vi "Waveform Processing Hub.vi"() -> ()   [LabVIEW 2014]
uses:
  <vilib>/Utility/file.llb/Write To Spreadsheet File (DBL).vi
  <vilib>/Utility/file.llb/Read From Spreadsheet File (DBL).vi
panel:
  in  "Baseline Pinch":bool
  in  "Orthogonal String Array Cluster":cluster{"Orthogonal String Array":string[]}={"Orthogonal String Array"=["1.1", "1.3", "1.5", "2.2", "2.4", "2.6", "2.8", "3.1", "3.3", "3.5", "3.7", "3.9", "4.4", "5.5", "6.8"]}
  in  "Empty String Array Cluster":cluster{"Empty String Array":string[]}
  in  "2-45 String Array Cluster":cluster{"2-45 String Array":string[]}={"2-45 String Array"=["2", "3", "4", "5", "6", "7", "8", "9", "10", "11", "12", "13", "14", "15", "16", "17", "18", "19", "20", "21", "22", "23", "24", "25", "26", "27", "28", "29", "30", "31", "32", "33", "34", "35", "36", "37", "38", "39", "40", "41", "42", "43", "44", "45"]}
  in  "1-5 String Array Cluster":cluster{"1-5 String Array":string[]}={"1-5 String Array"=["1", "2", "3", "4", "5"]}
  out "wfilter family":string="sym"
  out "MATLAB wfliter":string="sym5"
  out "Program Iterations":i32
  in  "Tab Control":T1(tab)
  out "Vertical Indicator":bool
  in  "Flip Vertically button":bool
  out "Horizontal Indicator":bool
  in  "Flip Horizontally Button":bool
  in  "Select File Type":string(combo)="Tab Delimited"
  out "Loaded File Data":dbl[][](graph)
  out "File Data":dbl[][](array[numeric])
  in  "Open Button":bool
  in  "Transpose":bool
  out "Transpose Indicator":bool
  out "Filtering Progress":u8(slide) scale=0.0..100.0
  out "Processed Spectra":dbl[][](graph)
  in  "Zero Data":bool
  in  "Normalize Data":bool
  out "File Data":dbl[][](graph)
  in  "Savitzy-Golay Filter":bool
  in  "Polynomial Order":i32=9
  in  "Side Points":i32=7
  in  "Play Button":bool
  in  "DWT BG Remove":bool
  in  "BG Remove Iterations":dbl=10.0
  in  "Wavelet #":string(combo)="5"
  in  "Wavelet Family":string(combo)="Symlets"
  in  "Process Spectra Separately":bool
  in  "Scale [>0]":dbl=8.0
  in  "DWT Filter":bool
  in  "# H-Freq Cuts":dbl=1.0
  in  "# L-Freq Cuts":dbl
  out "Zero & Normalized Data Out":dbl[][](array[numeric])
  in  "Save Button":bool
  out "File Data 2":dbl[][](graph)
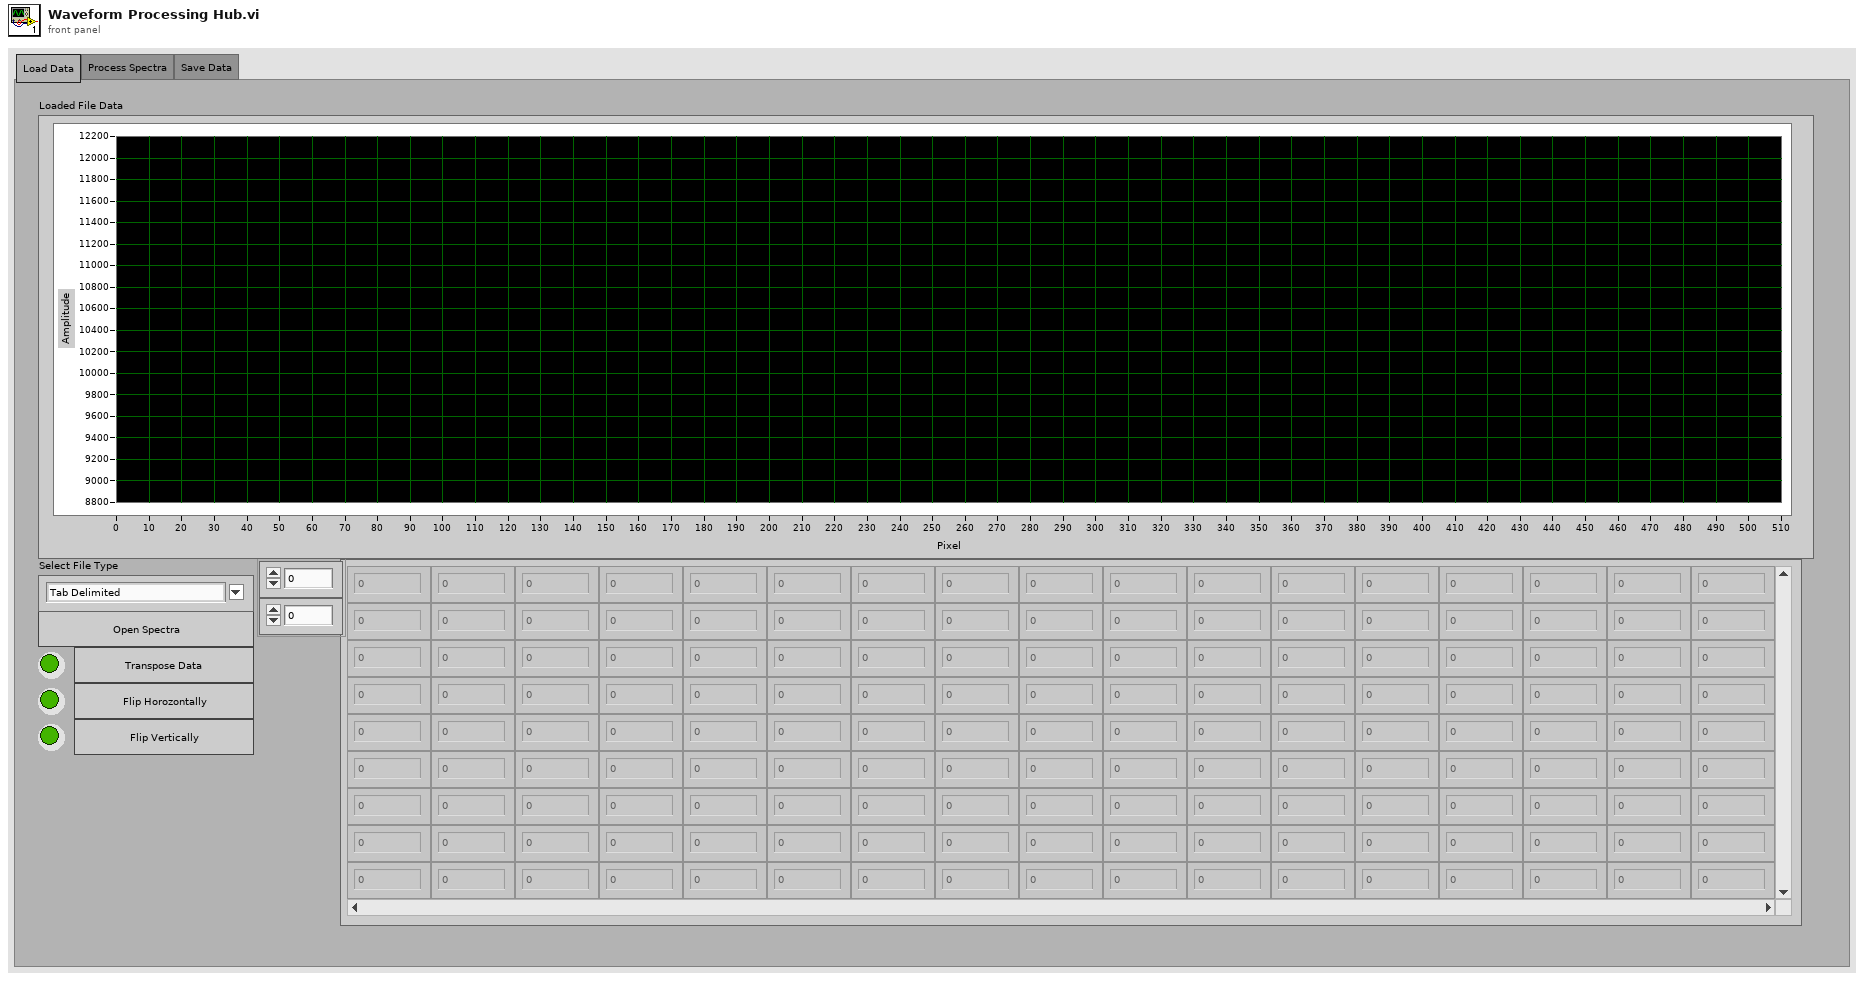
[diagram p1: front panel]
types:
  T1 = enum32{"Load Data", "Process Spectra", "Save Data"}
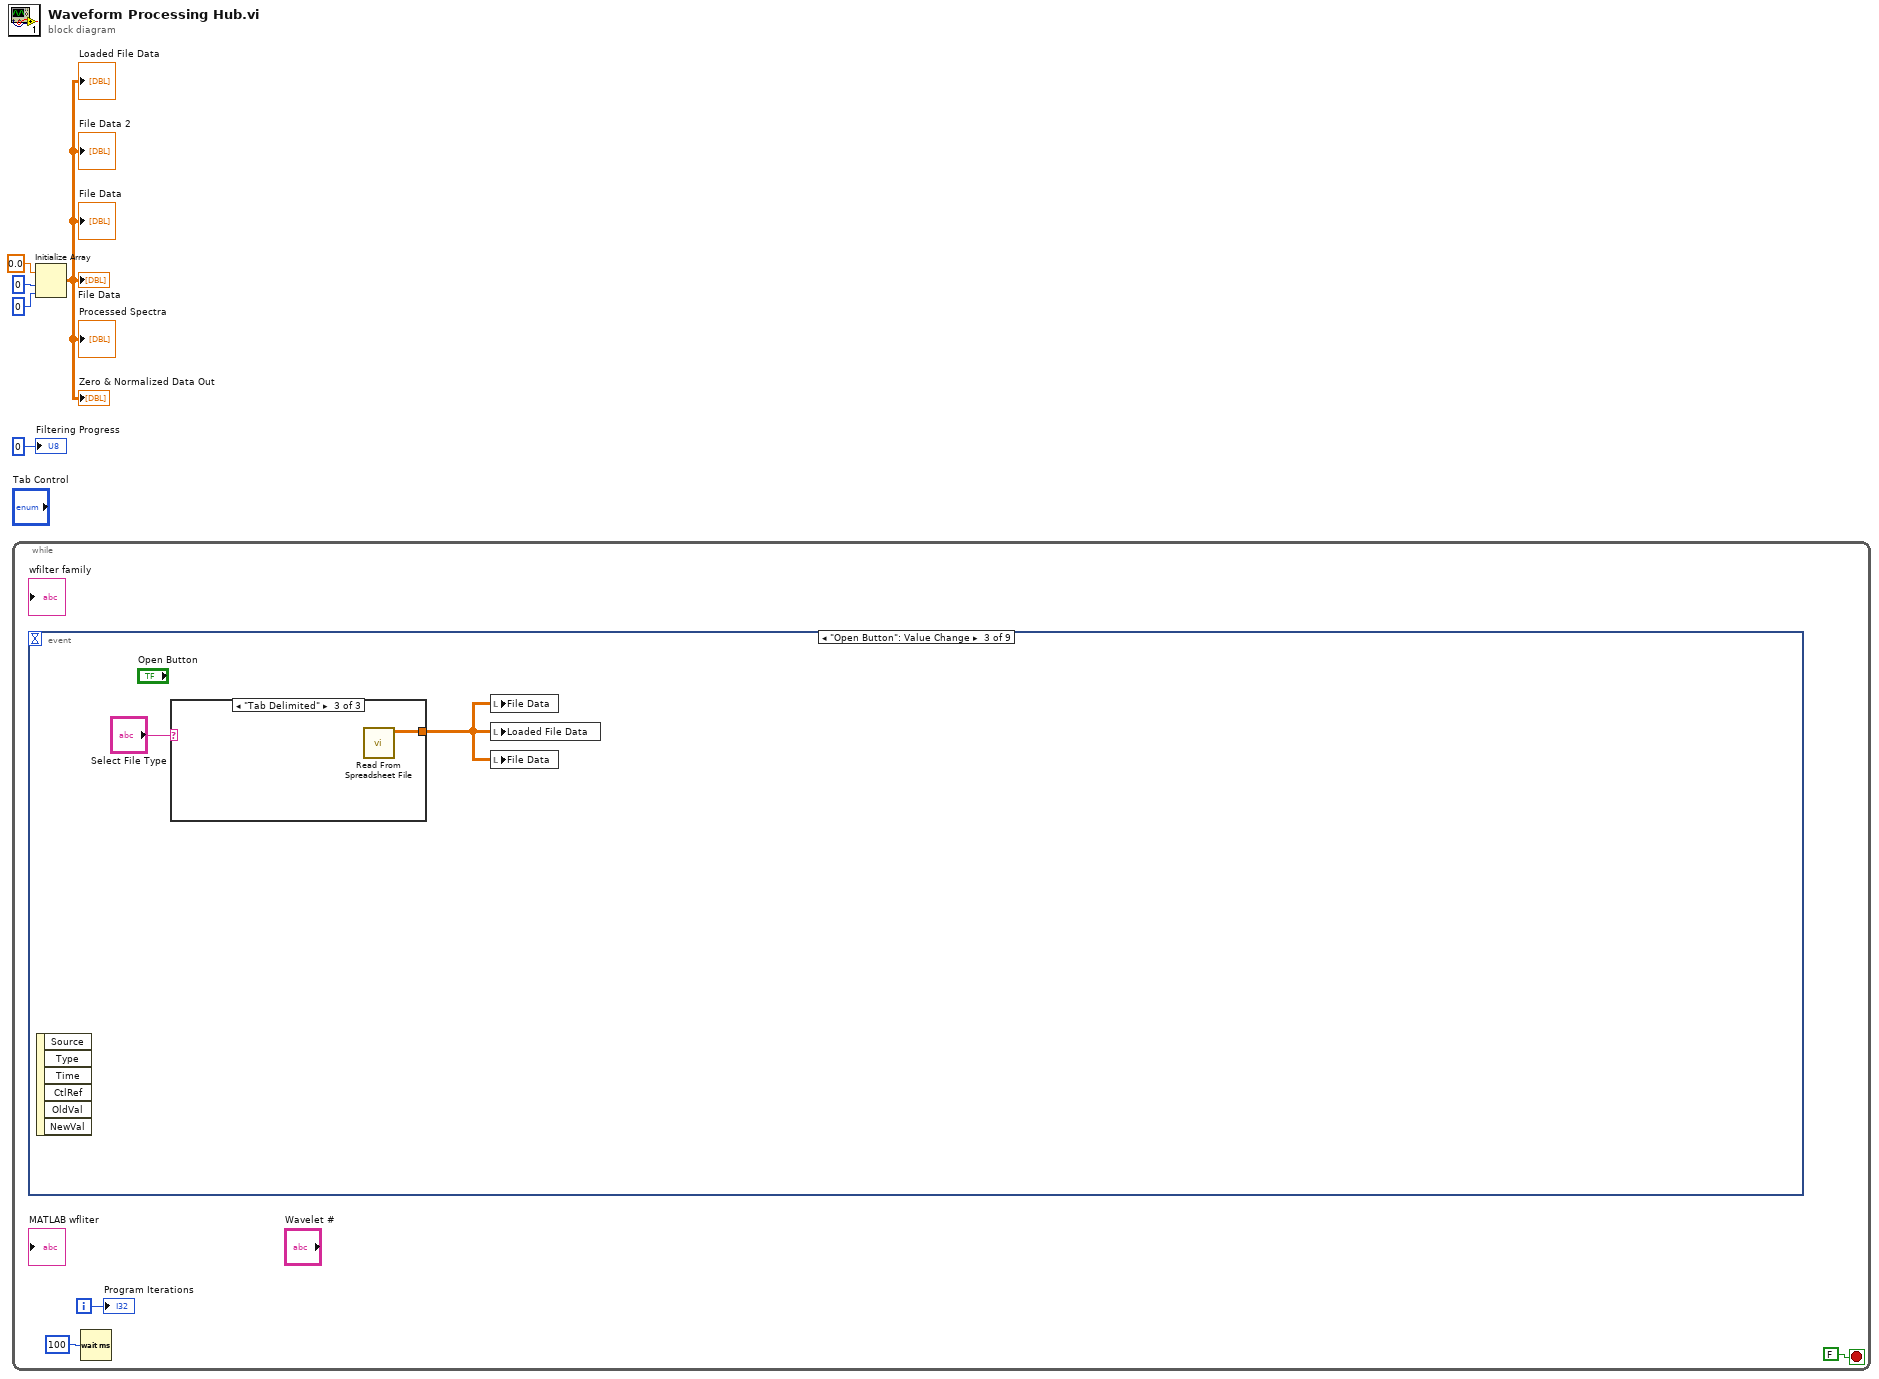
[diagram p0: block diagram]
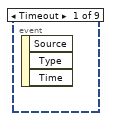
[diagram p2: hidden frame]
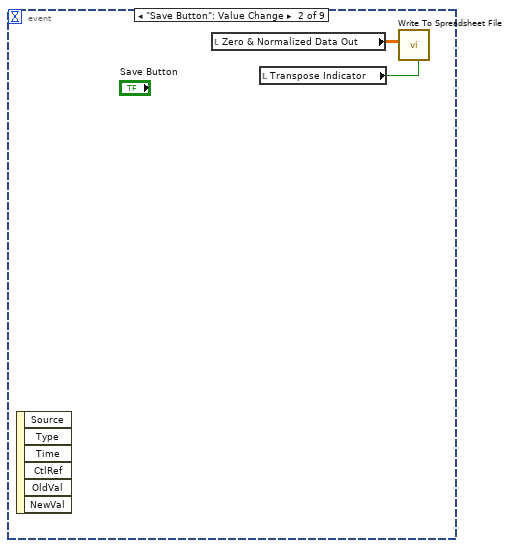
[diagram p3: hidden frame]
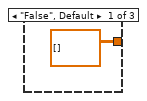
[diagram p4: hidden frame]
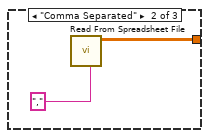
[diagram p5: hidden frame]
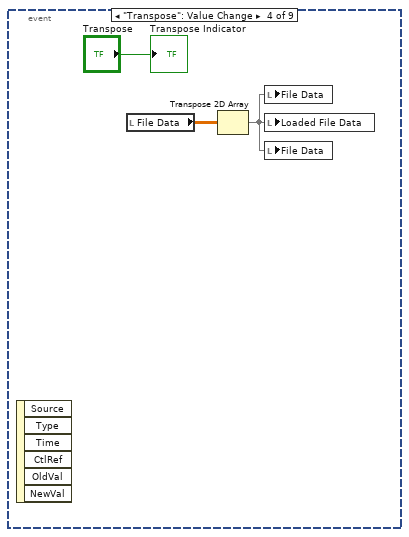
[diagram p6: hidden frame]
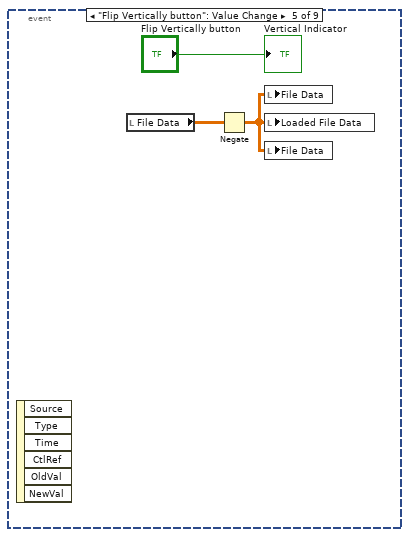
[diagram p7: hidden frame]
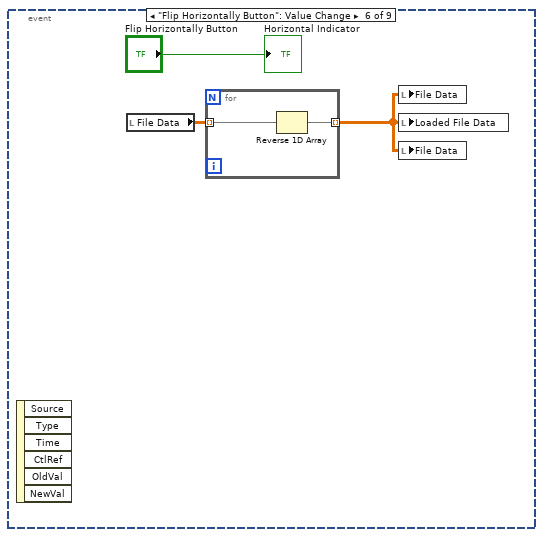
[diagram p8: hidden frame]
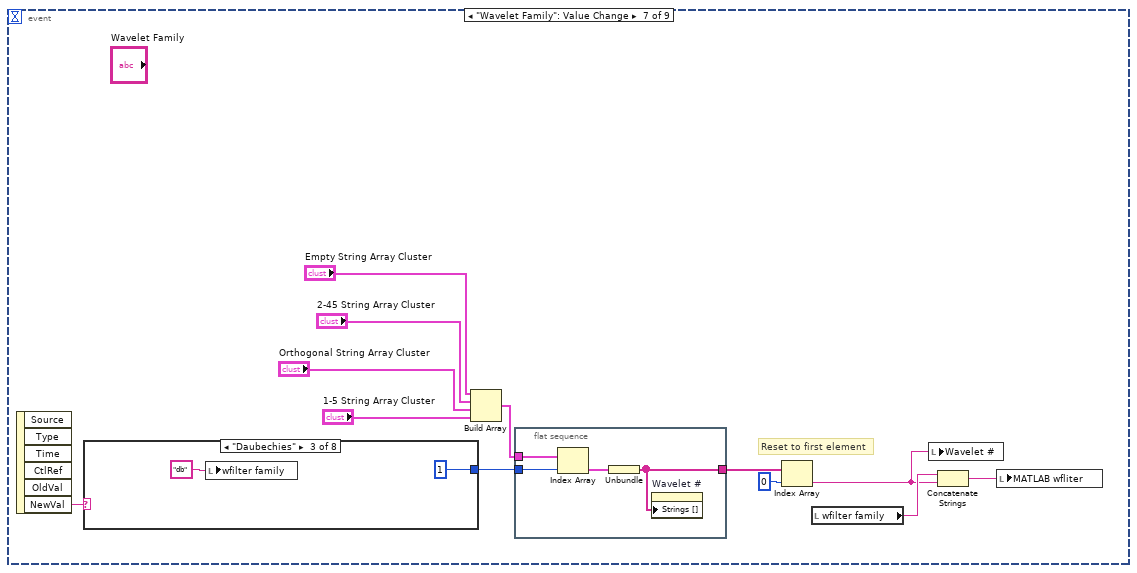
[diagram p9: hidden frame]
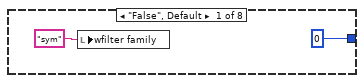
[diagram p10: hidden frame]
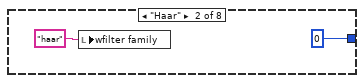
[diagram p11: hidden frame]
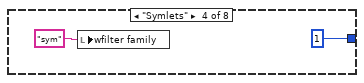
[diagram p12: hidden frame]
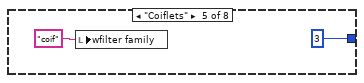
[diagram p13: hidden frame]
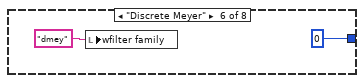
[diagram p14: hidden frame]
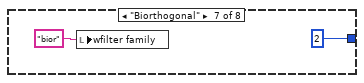
[diagram p15: hidden frame]
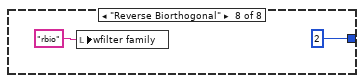
[diagram p16: hidden frame]
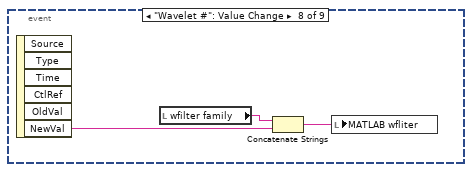
[diagram p17: hidden frame]
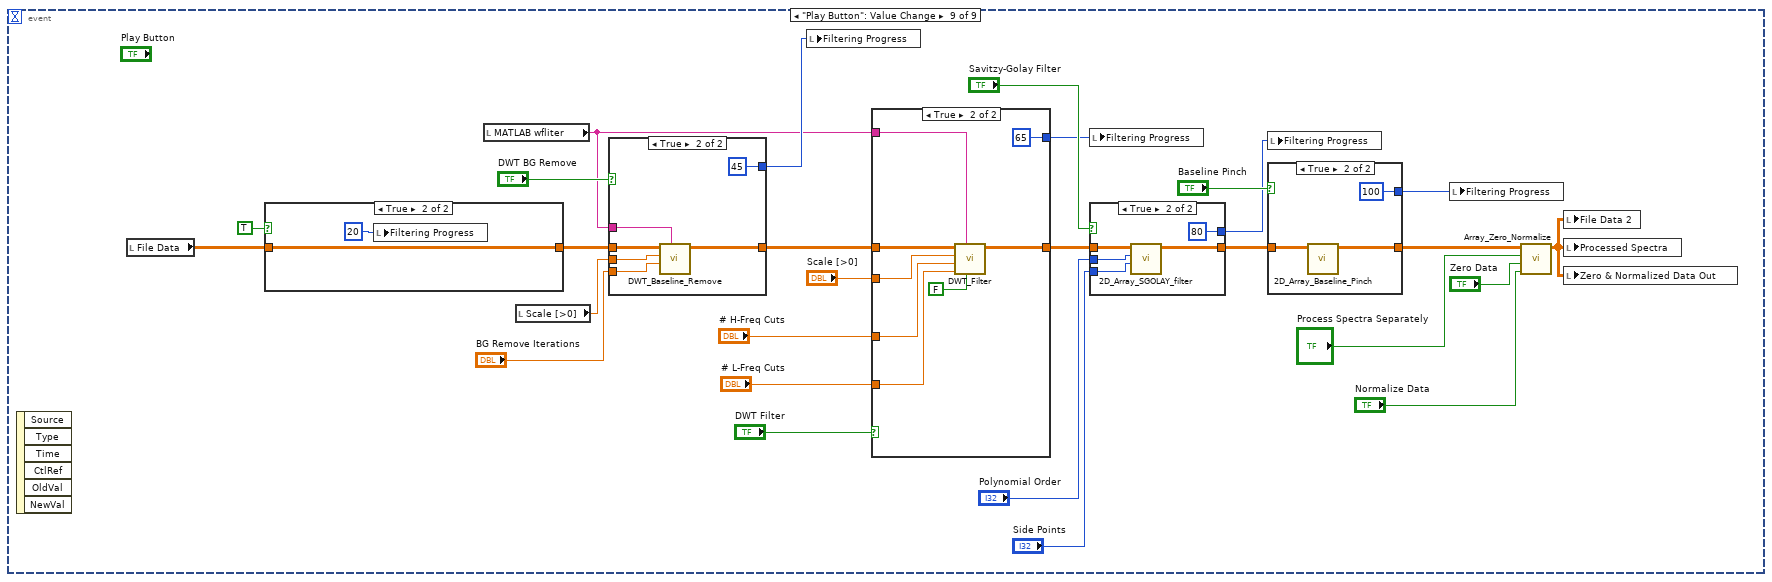
[diagram p18: hidden frame]
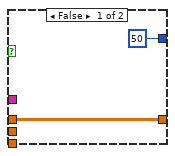
[diagram p20: hidden frame]
diagram:
  n1 = while {
    i -> [w7]
    stop <- FALSE stop-if-true
    n2 = event shown="[2] \"Open Button\": Value Change" {
      selector: _ -> [_ _ _ _ _ _ _ _ _]
      dyn-events: _ -> [_ _ _ _ _ _ _ _ _]
      timeout: _ -> [_ _ _ _ _ _ _ _ _]
      event Timeout {
        n3 = event-data() -> ()  [unwired: 1 in, 3 out]
      }
      event "Save Button": Value Change {
        n4 = event-data() -> ()  [unwired: 1 in, 6 out]
        n5 = local read "Zero & Normalized Data Out"() -> (w10:dbl[][])
        n6 = local read "Transpose Indicator"() -> (w9:bool)
        n7 = call-poly <vilib>:"Write To Spreadsheet File.vi"("transpose? (no:F)"=w9, "2D data"=w10) -> ()  [unwired: 6 in, 1 out]
      }
      event "Open Button": Value Change {
        n8 = event-data() -> ()  [unwired: 1 in, 6 out]
        n9 = case shown="\"Tab Delimited\"" "Select File Type" {
          tunnel: [dbl[][] [] ("all rows") w14 w16] -> w11
          frame "False", Default {
          }
          frame "Comma Separated" {
            n10 = call-poly <vilib>:"Read From Spreadsheet File.vi"("delimiter (\\t)"=",") -> ("all rows"=w14:dbl[][])  [unwired: 6 in, 4 out]
          }
          frame "Tab Delimited" {
            n11 = call-poly <vilib>:"Read From Spreadsheet File.vi"() -> ("all rows"=w16:dbl[][])  [unwired: 7 in, 4 out]
          }
        }
        n12 = local write "File Data"(w11) -> ()
        n13 = local write "Loaded File Data"(w11) -> ()
        n14 = local write "File Data"(w11) -> ()
      }
      event "Transpose": Value Change {
        n15 = event-data() -> ()  [unwired: 1 in, 6 out]
        n16 = local read "File Data"() -> (w18:dbl[][])
        n17 = Transpose 2D Array(2D array=w18) -> (transposed array=w17:dbl[][])
        n18 = local write "File Data"(w17) -> ()
        n19 = local write "Loaded File Data"(w17) -> ()
        n20 = local write "File Data"(w17) -> ()
        "Transpose Indicator" <- "Transpose"
      }
      event "Flip Vertically button": Value Change {
        n21 = event-data() -> ()  [unwired: 1 in, 6 out]
        n22 = local read "File Data"() -> (w21:dbl[][])
        n23 = Negate(x=w21) -> (-x=w20:dbl[][])
        n24 = local write "File Data"(w20) -> ()
        n25 = local write "Loaded File Data"(w20) -> ()
        n26 = local write "File Data"(w20) -> ()
        "Vertical Indicator" <- "Flip Vertically button"
      }
      event "Flip Horizontally Button": Value Change {
        n27 = event-data() -> ()  [unwired: 1 in, 6 out]
        n28 = local read "File Data"() -> (w24:dbl[][])
        n29 = for {
          tunnel: w24 -> [w27] mode=indexing
          tunnel: [w26] -> w23 mode=indexing
          n30 = Reverse 1D Array(array=w27) -> (reversed array=w26:dbl[])
        }
        n31 = local write "File Data"(w23) -> ()
        n32 = local write "Loaded File Data"(w23) -> ()
        n33 = local write "File Data"(w23) -> ()
        "Horizontal Indicator" <- "Flip Horizontally Button"
      }
      event "Wavelet Family": Value Change {
        # "Reset to first element"
        n34 = event-data() -> ("NewVal"=w28:string)  [unwired: 1 in, 5 out]
        n35 = case shown="\"Daubechies\"" w28 {
          tunnel: [0 0 1 1 3 0 2 2] -> w36
          frame "False", Default {
            n36 = local write "wfilter family"("sym" ("wfilter family")) -> ()
          }
          frame "Haar" {
            n37 = local write "wfilter family"("haar" ("MATLAB wfilter")) -> ()
          }
          frame "Daubechies" {
            n38 = local write "wfilter family"("db" ("wfilter family")) -> ()
          }
          frame "Symlets" {
            n39 = local write "wfilter family"("sym" ("wfilter family")) -> ()
          }
          frame "Coiflets" {
            n40 = local write "wfilter family"("coif" ("wfilter family")) -> ()
          }
          frame "Discrete Meyer" {
            n41 = local write "wfilter family"("dmey" ("wfilter family")) -> ()
          }
          frame "Biorthogonal" {
            n42 = local write "wfilter family"("bior" ("wfilter family")) -> ()
          }
          frame "Reverse Biorthogonal" {
            n43 = local write "wfilter family"("rbio" ("wfilter family")) -> ()
          }
        }
        n44 = Build Array("Empty String Array Cluster", "2-45 String Array Cluster", "Orthogonal String Array Cluster", "1-5 String Array Cluster") -> (w29:cluster{"1-5 String Array":string[]}[])
        n45 = flat-sequence {
          tunnel: w29 -> [w59]
          tunnel: [w57] -> w34
          tunnel: w36 -> [w56]
          frame #0 {
            n46 = Index Array(array=w59, index=w56) -> (element=w58:cluster{"1-5 String Array":string[]})
            n47 = Unbundle(w58) -> ("1-5 String Array"=w57:string[])
            n48 = property on="Wavelet #" class="CmbBox"("Strings []"=w57) -> ()  [unwired: 2 in, 2 out]
          }
        }
        n49 = Index Array(array=w34, index=0) -> (element=w38:string)
        n50 = local read "wfilter family"() -> (w39:string)
        n51 = local write "Wavelet #"(w38) -> ()
        n52 = Concatenate Strings(w39, w38) -> (w37:string)
        n53 = local write "MATLAB wfliter"(w37) -> ()
      }
      event "Wavelet #": Value Change {
        n54 = event-data() -> ("NewVal"=w60:string)  [unwired: 1 in, 5 out]
        n55 = local read "wfilter family"() -> (w62:string)
        n56 = Concatenate Strings(w62, w60) -> (w61:string)
        n57 = local write "MATLAB wfliter"(w61) -> ()
      }
      event "Play Button": Value Change {
        n58 = event-data() -> ()  [unwired: 1 in, 6 out]
        n59 = local read "File Data"() -> (w75:dbl[][])
        n60 = case shown="True" TRUE {
          tunnel: w75 -> [w90 w92]
          tunnel: [w90 w92] -> w68
          frame False {
          }
          frame True {
            n61 = local write "Filtering Progress"(u8 20 ("Filtering Progress")) -> ()
          }
        }
        n62 = local read "MATLAB wfliter"() -> (w63:string)
        n63 = local read "Scale [>0]"() -> (w78:dbl)
        n64 = case shown="True" "DWT BG Remove" {
          tunnel: w68 -> [w94 w100]
          tunnel: w78 -> [_ w98]
          tunnel: "BG Remove Iterations" -> [_ w99]
          tunnel: [w94 w97] -> w67
          tunnel: [u8 50 ("Filtering Progress") u8 45 ("Filtering Progress")] -> w65
          tunnel: w63 -> [_ w95]
          frame False {
          }
          frame True {
            n65 = call "DWT_Baseline_Remove.vi"("String"=w95, "DWT Iterations"=w99, "Scale [>0]"=w98, "File Data In 2"=w100) -> ("2-D Array of Real"=w97:dbl[][])  [unwired: 7 in]
          }
        }
        n66 = local write "Filtering Progress"(w65) -> ()
        n67 = case shown="True" "DWT Filter" {
          tunnel: w67 -> [w102 w110]
          tunnel: "# L-Freq Cuts" -> [_ w109]
          tunnel: "# H-Freq Cuts" -> [_ w108]
          tunnel: "Scale [>0]" -> [_ w107]
          tunnel: [w102 w106] -> w66
          tunnel: [u8 20 ("Filtering Progress") u8 65 ("Filtering Progress")] -> w64
          tunnel: w63 -> [_ w104]
          frame False {
          }
          frame True {
            n68 = call "DWT_Filter.vi"("Remove nth Approximation"=FALSE, "String"=w104, "# Lfreq Wavelets to Cut"=w109, "# Hfreq Wavelets to Cut"=w108, "Scale [>0]"=w107, "File Data In 2"=w110) -> ("2-D Array of Real"=w106:dbl[][])  [unwired: 5 in]
          }
        }
        n69 = local write "Filtering Progress"(w64) -> ()
        n70 = case shown="True" "Savitzy-Golay Filter" {
          tunnel: [w112 w117] -> w70
          tunnel: "Polynomial Order" -> [_ w116]
          tunnel: "Side Points" -> [_ w115]
          tunnel: w66 -> [w112 w114]
          tunnel: [u8 65 ("Filtering Progress") u8 80 ("Filtering Progress")] -> w72
          frame False {
          }
          frame True {
            n71 = call "2D_Array_SGOLAY_filter.vi"("side points"=w115, "polynomial order"=w116, "File Data In"=w114) -> ("File Data In 2"=w117:dbl[][])  [unwired: 8 in]
          }
        }
        n72 = local write "Filtering Progress"(w72) -> ()
        n73 = case shown="True" "Baseline Pinch" {
          tunnel: w70 -> [w119 w122]
          tunnel: [w119 w121] -> w69
          tunnel: [u8 100 ("Filtering Progress") u8 100 ("Filtering Progress")] -> w71
          frame False {
          }
          frame True {
            n74 = call "2D_Array_Baseline_Pinch.vi"("Data In"=w122) -> ("Pinched Data Out"=w121:dbl[][])  [unwired: 10 in]
          }
        }
        n75 = local write "Filtering Progress"(w71) -> ()
        n76 = call "Array_Zero_Normalize.vi"("Normalize Data"="Normalize Data", "Zero Data"="Zero Data", "Process Rows Seperately"="Process Spectra Separately", "x+y"=w69) -> ("Normalized Array Out"=w74:dbl[][])  [unwired: 5 in, 2 out]
        n77 = local write "File Data 2"(w74) -> ()
        n78 = local write "Processed Spectra"(w74) -> ()
        n79 = local write "Zero & Normalized Data Out"(w74) -> ()
      }
    }
    n80 = Wait (ms)(milliseconds to wait=u32 100) -> ()  [unwired: 1 out]
    "Program Iterations" <- w7
  }
  n81 = Initialize Array(0.0 ("element"), 0 ("dimension size"), 0 ("dimension size")) -> (→"File Data" →"Zero & Normalized Data Out" →"File Data" →"Processed Spectra" →"File Data 2" →"Loaded File Data":dbl[][])
  "Filtering Progress" <- u8 0 ("Filtering Progress")
